vi "Get_MeasurementsII.vi"(0 "VISA resource name":refnum<visa-resource-name>="Oscilloscope", 1 "Amplitude IN":dbl=0.25, 4 "Attenuation":i32, 5 "Measurements per channel":i32=5, 6 "Clipping":i32, 7 "Fine Clipping":i32, 8 "Amplitude":bool=TRUE, 9 "file path (dialog if empty)":path=path "F:/L0_Measurements_291014_174904.txt", 12 "Width":bool=TRUE, 13 "Write to a file?":bool, 14 "ASIC Channel":i32, 15 "error in":errorcluster, 16 "Delay":bool=TRUE, 17 "Oscilloscope Channel":i32(ring)=1 items=["Channel 1"=1, "Channel 2"=2, "Channel 3"=3, "Channel 4"=4, "Function 1"=5, "Function 2"=6, "Function 3"=7, "Function 4"=8, "Memory 1"=9, "Memory 2"=10, "Memory 3"=11, "Memory 4"=12]) -> (20 "VISA resource name out":refnum<visa-resource-name>="Oscilloscope", 21 "Vpp_Array":dbl[](array[numeric]), 23 "Width Array":dbl[](array[numeric]), 25 "Setup_Time_Array":dbl[](array[numeric]), 27 "error out":errorcluster)   [LabVIEW 2012]
uses:
  <vilib>/Utility/file.llb/Write To Spreadsheet File (string).vi
panel:
  out "new file path (Not A Path if cancelled)":path=path "F:/L0_Measurements_291014_174904.txt"
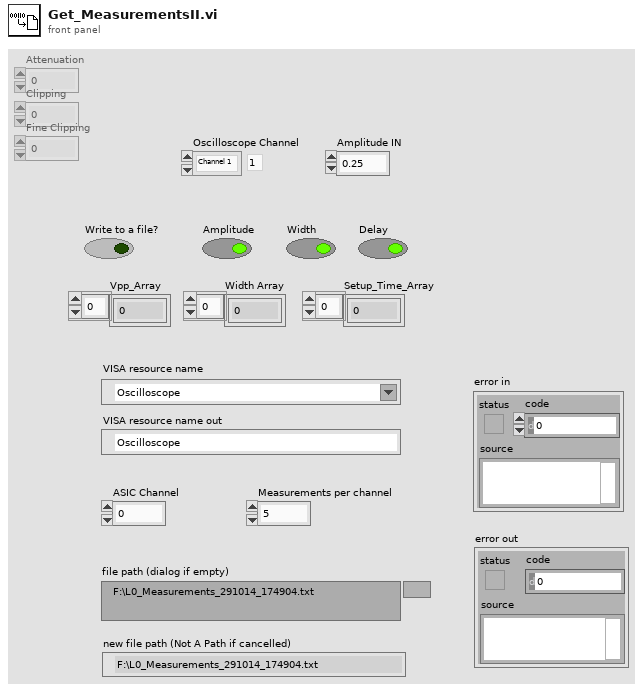
[diagram p1: front panel]
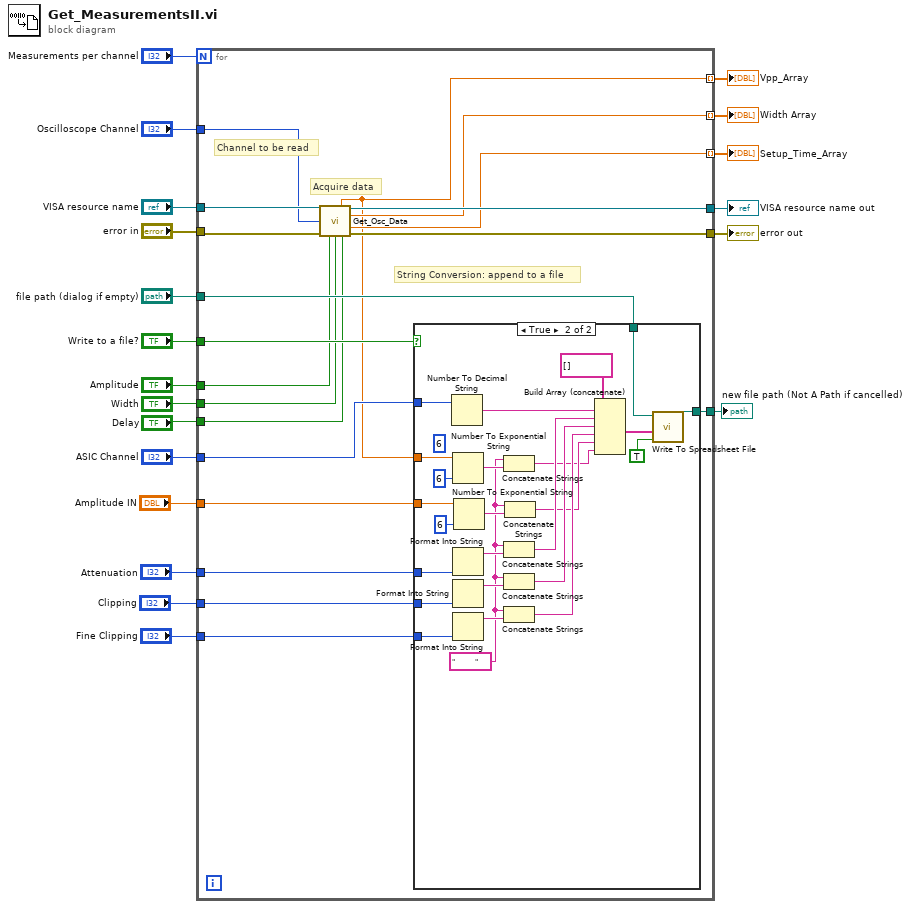
[diagram p0: block diagram]
diagram:
  n1 = for {
    N: "Measurements per channel" -> [_]
    tunnel: "VISA resource name" -> [w39]
    tunnel: "error in" -> [w38]
    tunnel: "ASIC Channel" -> [w33]
    tunnel: "file path (dialog if empty)" -> [w35]
    tunnel: [w37] -> w15
    tunnel: [w36] -> w12
    tunnel: [w34] -> w14
    tunnel: [w22] -> w13 mode=indexing
    tunnel: [w32] -> w11 mode=indexing
    tunnel: [w23] -> w10 mode=indexing
    tunnel: "Write to a file?" -> [w31]
    tunnel: "Amplitude" -> [w30]
    tunnel: "Width" -> [w29]
    tunnel: "Delay" -> [w28]
    tunnel: "Oscilloscope Channel" -> [w27]
    tunnel: "Attenuation" -> [w26]
    tunnel: "Clipping" -> [w25]
    tunnel: "Fine Clipping" -> [w24]
    tunnel: "Amplitude IN" -> [w21]
    # "Acquire data"
    # "Channel to be read"
    # "String Conversion: append to a file"
    n2 = call "Get_Osc_Data.vi"("VISA resource name"=w39, "Channel"=w27, "error in"=w38, "Amplitude"=w30, "Width"=w29, "Delay"=w28) -> ("Amplitude"=w22:dbl, "VISA resource name out"=w37:refnum<visa-resource-name>, "Width Pos"=w32:dbl, "Delay"=w23:dbl, "error out"=w36:errorcluster)  [unwired: 4 in, 1 out]
    n3 = case shown="True" w31 {
      tunnel: w35 -> [w40 w61]
      tunnel: [w40 w60] -> w34
      tunnel: w33 -> [_ w59]
      tunnel: w22 -> [_ w58]
      tunnel: w26 -> [_ w57]
      tunnel: w25 -> [_ w56]
      tunnel: w24 -> [_ w55]
      tunnel: w21 -> [_ w44]
      frame False {
      }
      frame True {
        w45 = "          "
        (unwired) i16 6 ("precision (6)")
        n4 = Number To Decimal String(number=w59) -> (decimal integer string=w41:string)  [unwired: 1 in]
        n5 = Number To Exponential String(number=w58, precision (6)=i16 6) -> (E-format string=w51:string)  [unwired: 2 in]
        n6 = Format Into String(w57) -> (resulting string=w54:string)  [unwired: 3 in, 1 out]
        n7 = Format Into String(w56) -> (resulting string=w53:string)  [unwired: 3 in, 1 out]
        n8 = Format Into String(w55) -> (resulting string=w52:string)  [unwired: 3 in, 1 out]
        n9 = Number To Exponential String(number=w44, precision (6)=i16 6) -> (E-format string=w46:string)  [unwired: 2 in]
        n10 = Concatenate Strings(w45, w51) -> (w42:string)
        n11 = Concatenate Strings(w45, w54) -> (w50:string)
        n12 = Concatenate Strings(w45, w53) -> (w49:string)
        n13 = Concatenate Strings(w45, w52) -> (w48:string)
        n14 = Concatenate Strings(w45, w46) -> (w43:string)
        n15 = Build Array (concatenate)(string[] [] ("array"), w41, w50, w49, w48, w43, w42) -> (w64:string[])
        n16 = call-poly <vilib>:"Write To Spreadsheet File.vi"("append to file? (new file:F)"=TRUE, "1D data"=w64, "file path (dialog if empty)"=w61) -> ("new file path (Not A Path if cancelled)"=w60:path)  [unwired: 5 in]
      }
    }
  }
  "VISA resource name out" <- w15
  "error out" <- w12
  "new file path (Not A Path if cancelled)" <- w14
  "Vpp_Array" <- w13
  "Width Array" <- w11
  "Setup_Time_Array" <- w10
